vi "Simultaneous Start with Hardware Trigger.vi"() -> ()   [LabVIEW 2009]
uses:
  <vilib>/DAQmx/write.llb/DAQmx Write (Analog Wfm 1Chan NSamp).vi
  <vilib>/DAQmx/configure/timing.llb/DAQmx Timing (Sample Clock).vi
  <vilib>/DAQmx/configure/trigger.llb/DAQmx Start Trigger (Digital Edge).vi
  <vilib>/DAQmx/create/channels.llb/DAQmx Create Channel (AO-Voltage-Basic).vi
  <vilib>/DAQmx/create/channels.llb/DAQmx Create Channel (AI-Voltage-Basic).vi
  <vilib>/DAQmx/read.llb/DAQmx Read (Analog 1D DBL 1Chan NSamp).vi
  Program Files/National Instruments/LabVIEW 2009/resource/objmgr/daqmx.rc
  <vilib>/measure/NI_MABase.lvlib
panel:
  out "data":dbl[](graph)
  out "signal out":waveform(dbl)(graph)
  in  "stop":bool
  in  "input rate":dbl=1000.0 format="%0.2f"
  in  "output rate":dbl(slide)=1000.0 scale=100.0..2000.0
  in  "AI channel":tag="Dev1/ai2"
  in  "AO channel":tag="Dev1/ao0"
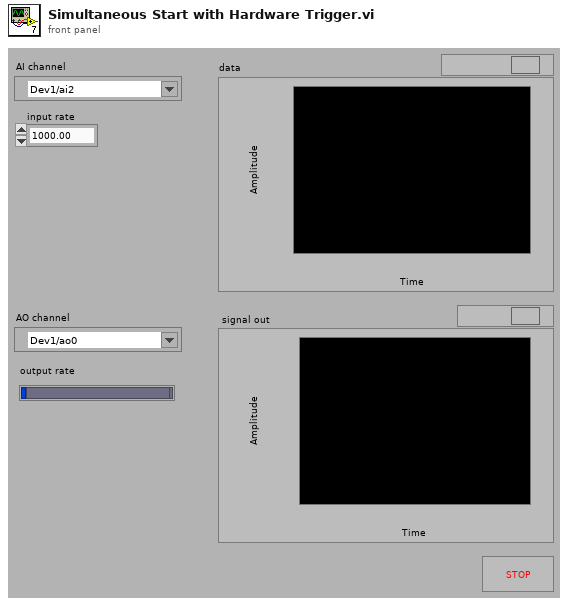
[diagram p1: front panel]
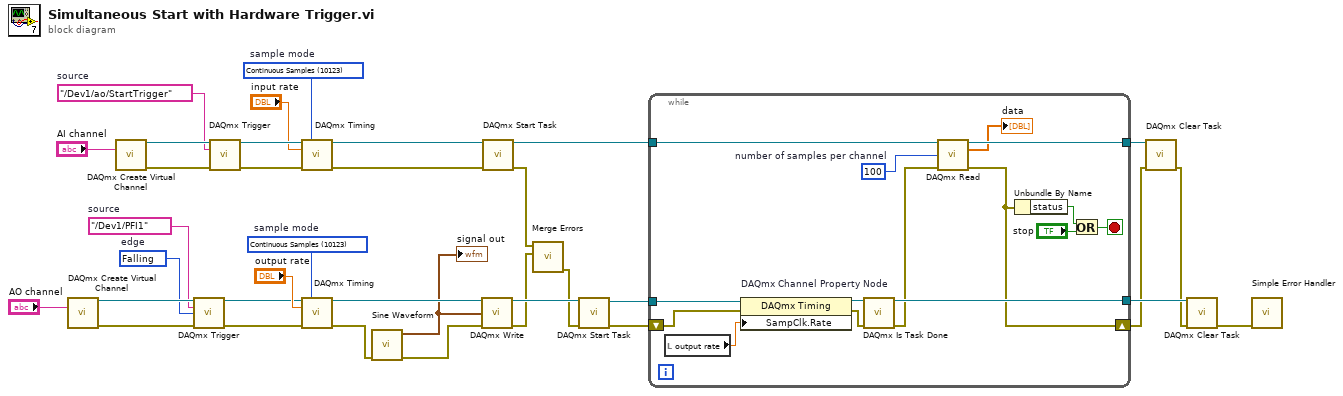
[diagram p0: block diagram]
diagram:
  w1 = 10171 items=["Rising"=10280, "Falling"=10171]  # edge
  w2 = tag "/Dev1/PFI1"  # source
  w12 = tag "/Dev1/ao/StartTrigger"  # source
  w13 = 10123 items=["Finite Samples"=10178, "Continuous Samples"=10123, "Hardware Timed Single Point"=12522]  # sample mode
  w14 = 10123 items=["Finite Samples"=10178, "Continuous Samples"=10123, "Hardware Timed Single Point"=12522]  # sample mode
  n1 = call-poly <vilib>:"DAQmx Create Virtual Channel.vi"("physical channels"="AO channel") -> ("task out"=w6:refnum<k21>, "error out"=w4:errorcluster)  [unwired: 13 in]
  n2 = call-poly <vilib>:"DAQmx Create Virtual Channel.vi"("physical channels"="AI channel") -> ("task out"=w31:refnum<k21>, "error out"=w35:errorcluster)  [unwired: 13 in]
  n3 = call-poly <vilib>:"DAQmx Trigger.vi"("task/channels in"=w6, "source"=w2, "edge"=w1, "error in"=w4) -> ("task out"=w5:refnum<k21>, "error out"=w3:errorcluster)  [unwired: 10 in]
  n4 = call-poly <vilib>:"DAQmx Trigger.vi"("task/channels in"=w31, "source"=w12, "error in"=w35) -> ("task out"=w26:refnum<k21>, "error out"=w24:errorcluster)  [unwired: 11 in]
  n5 = call-poly <vilib>:"DAQmx Timing.vi"("task/channels in"=w26, "sample mode"=w14, "rate"="input rate", "error in"=w24) -> ("task out"=w25:refnum<k21>, "error out"=w7:errorcluster)  [unwired: 10 in]
  n6 = call-poly <vilib>:"DAQmx Timing.vi"("task/channels in"=w5, "sample mode"=w13, "rate"="output rate", "error in"=w3) -> ("task out"=w23:refnum<k21>, "error out"=w17:errorcluster)  [unwired: 10 in]
  n7 = call <vilib>:"Sine Waveform.vi"("error in (no error)"=w17) -> ("error out"=w16:errorcluster, "signal out"=w15:waveform(dbl))  [unwired: 9 in]
  "signal out" <- w15
  n8 = call-poly <vilib>:"DAQmx Write.vi"("task/channels in"=w23, "data"=w15, "error in"=w16) -> ("task out"=w32:refnum<k21>, "error out"=w9:errorcluster)  [unwired: 10 in, 1 out]
  n9 = call <vilib>:"DAQmx Start Task.vi"("task/channels in"=w25, "error in"=w7) -> ("task out"=w30:refnum<k21>, "error out"=w8:errorcluster)  [unwired: 12 in]
  n10 = call <vilib>:"Merge Errors.vi"("error in 2 (no error)"=w9, "error in 1 (no error)"=w8) -> ("error out"=w10:errorcluster)  [unwired: 5 in]
  n11 = call <vilib>:"DAQmx Start Task.vi"("task/channels in"=w32, "error in"=w10) -> ("task out"=w33:refnum<k21>, "error out"=w11:errorcluster)  [unwired: 12 in]
  n12 = while {
    tunnel: [w49] -> w34
    tunnel: w33 -> [w47]
    tunnel: w30 -> [w46]
    tunnel: [w45] -> w29
    shift-right: [w43] -> w20
    shift-left: w11 -> [w37]
    stop <- w40 stop-if-true
    w38 = 100  # number of samples per channel
    n13 = local read "output rate"() -> (w39:dbl)
    n14 = property on="DAQmx Channel Property Node" class="DAQmx Timing"(reference=w47, error in=w37, "SampClk.Rate"=w39) -> (reference out=w48:refnum<k21>, error out=w50:errorcluster)
    n15 = call <vilib>:"DAQmx Is Task Done.vi"("task/channels in"=w48, "error in"=w50) -> ("task out"=w49:refnum<k21>, "error out"=w44:errorcluster)  [unwired: 11 in, 1 out]
    n16 = call-poly <vilib>:"DAQmx Read.vi"("task/channels in"=w46, "number of samples per channel"=w38, "error in"=w44) -> ("task out"=w45:refnum<k21>, "data"=→"data":dbl[], "error out"=w43:errorcluster)  [unwired: 10 in]
    n17 = Unbundle By Name "Unbundle By Name"(w43) -> ("status"=w42:bool)
    n18 = Or(x=w42, y="stop") -> (x .or. y?=w40:bool)
  }
  n19 = call <vilib>:"DAQmx Clear Task.vi"("task in"=w29, "error in"=w20) -> ("error out"=w19:errorcluster)  [unwired: 13 in]
  n20 = call <vilib>:"DAQmx Clear Task.vi"("task in"=w34, "error in"=w19) -> ("error out"=w18:errorcluster)  [unwired: 13 in]
  n21 = call <vilib>:"Simple Error Handler.vi"("error in (no error)"=w18) -> ()  [unwired: 4 in, 5 out]
